vi "Phasor Compute Gated Decay (Tolerance).vi"(4 "Non Dirac IRF or non-0 lifetime":bool, 6 "tolerance":dbl, 8 "Error In":errorcluster, 9 "IRF Period":dbl, 10 "Gate & Decay Parameters Array":T1[](array[typedef]) {"A" format="%#_4g"; "s" format="%#_4g"; "sF" format="%#_4g"; "sR" format="%#_4g"; "t_i" format="%#_4g"; "t_0" format="%#_4g"; "tau" format="%#_4g"; "T" format="%#_4g"; "W" format="%#_4g"}, 11 "Time Points {t_i}":dbl[](array[numeric])) -> (0 "Error Out":errorcluster, 3 "{F(t_i)}":dbl[](array[numeric]))   [LabVIEW 2021, in "Phasor.lvlib"]
uses:
  Phasor.lvlib
  Phasor Gate & Decay Parameters.ctl
  Phasor Gate Type.ctl
  Phasor IRF Model.ctl
  Graphs/XY Graph/XY Graph Plot Data.ctl
  Phasor Abort Parallel Computation.vi
  1D Quadrature Integrand for Gated Decay.vi
  <vilib>/Utility/error.llb/Error Cluster From Error Code.vi
  <vilib>/ErrorRing/Error Ring.xnode
  Math/Math.lvlib
  Utilities/Utilities.lvlib
  Graphs/XY Graph/XY Graph Add-Ons.lvlib
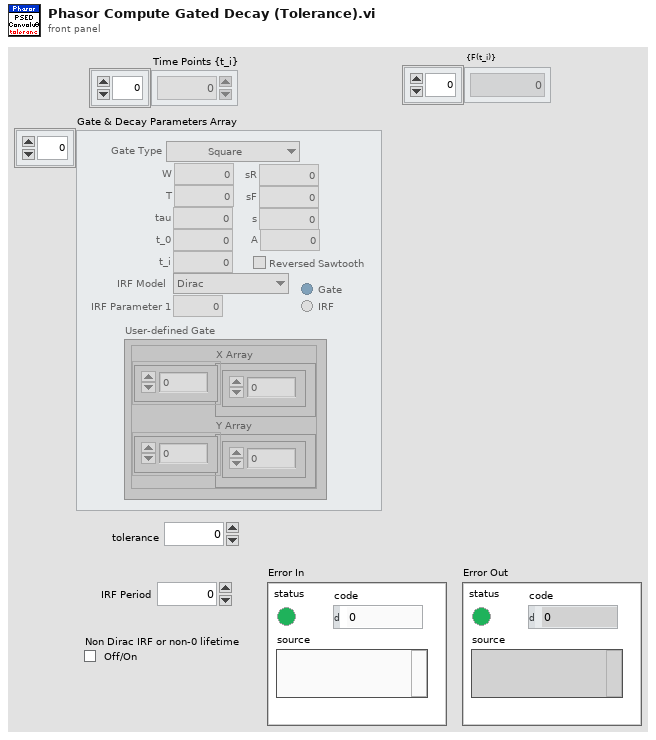
[diagram p1: front panel]
types:
  T1 = typedef "Phasor.lvlib/Phasor Gate & Decay Parameters.ctl" = cluster{"W":dbl, "T":dbl, "tau":dbl, "t_0":dbl, "Gate Type":T2, "t_i":dbl, "sR":dbl, "sF":dbl, "s":dbl, "Reversed Sawtooth":bool, "IRF Model":T3, "IRF Parameter 1":dbl, "User-defined Gate":T4, "Type of User-defined Function":enum32{"Gate", "IRF"}, "A":dbl}
  T2 = typedef "Phasor.lvlib/Phasor Gate Type.ctl" = enum16{"Square", "Finite Edge Square", "Finite Edge, Tilted Top Square", "Triangle", "Sawtooth", "User-defined"}
  T3 = typedef "Phasor.lvlib/Phasor IRF Model.ctl" = enum16{"Dirac", "Exponential"}
  T4 = typedef "XY Graph Add-Ons.lvlib/XY Graph Plot Data.ctl" = cluster{"X Array":dbl[], "Y Array":dbl[]}
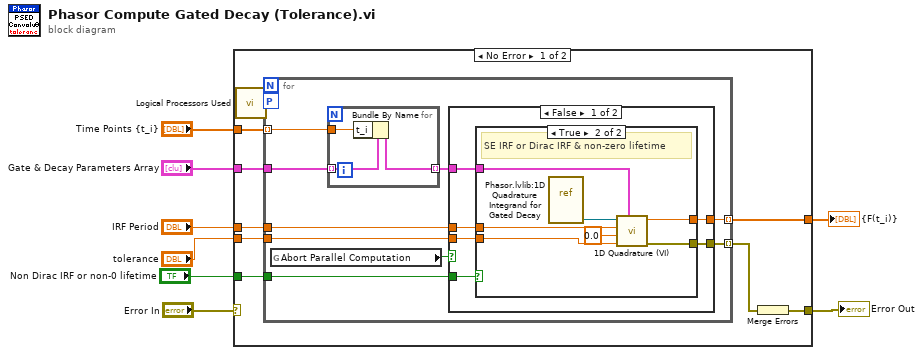
[diagram p0: block diagram]
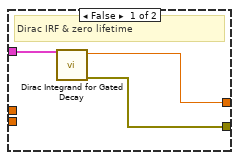
[diagram p2: hidden frame]
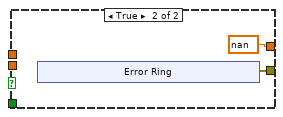
[diagram p3: hidden frame]
diagram:
  n1 = case shown="No Error" "Error In" {
    selector: "Error In" -> [_ w52]
    tunnel: "Non Dirac IRF or non-0 lifetime" -> [w17 _]
    tunnel: "IRF Period" -> [w16 _]
    tunnel: "tolerance" -> [w15 _]
    tunnel: [w14 _] -> w5
    tunnel: "Gate & Decay Parameters Array" -> [w13 _]
    tunnel: "Time Points {t_i}" -> [w12 _]
    tunnel: [w10 w52] -> w1
    frame No Error {
      n2 = call "Logical Processors Used.vi"() -> ("# Logical Processor Used"=w9:i32)  [unwired: 6 in]
      n3 = for {
        tunnel: w12 -> [w22] mode=indexing
        tunnel: w13 -> [w21]
        tunnel: [w26] -> w14 mode=indexing
        workers-P: w9 -> [_]
        tunnel: [w24] -> w11 mode=indexing
        tunnel: w15 -> [w25]
        tunnel: w16 -> [w23]
        tunnel: w17 -> [w19]
        n4 = global read "Phasor Abort Parallel Computation.vi" "Abort Parallel Computation"() -> (w18:bool)
        n5 = for {
          tunnel: w22 -> [w51]
          tunnel: w21 -> [w50] mode=indexing
          tunnel: [w49] -> w20 mode=indexing
          n6 = Bundle By Name(cluster=w50, "t_i"=w51) -> (w49:T1)
        }
        n7 = case shown="False" w18 {
          tunnel: w20 -> [w32 _]
          tunnel: [w31 nan ("result")] -> w26
          tunnel: [w30 w43] -> w24
          tunnel: w25 -> [w29 _]
          tunnel: w23 -> [w28 _]
          tunnel: w19 -> [w27 _]
          frame False {
            n8 = case shown="True" w27 {
              tunnel: [w34 w42] -> w31
              tunnel: w32 -> [w35 w41]
              tunnel: [w33 w40] -> w30
              tunnel: w29 -> [_ w39]
              tunnel: w28 -> [_ w37]
              frame False {
                # "Dirac IRF & zero lifetime"
                n9 = call "Dirac Integrand for Gated Decay.vi"("data"=w35) -> ("Error Out"=w33:errorcluster, "F(X)"=w34:dbl)  [unwired: 9 in]
              }
              frame True {
                # "SE IRF or Dirac IRF & non-zero lifetime"
                n10 = vi-ref "Phasor.lvlib:1D Quadrature Integrand for Gated Decay.vi"() -> (w36:refnum<vi>)
                n11 = call "1D Quadrature (VI).vi"("data"=w41, "tolerance"=w39, "lower limit"=0.0, "upper limit"=w37, "integrand"=w36) -> ("Error Out"=w40:errorcluster, "result"=w42:dbl)  [unwired: 5 in]
              }
            }
          }
          frame True {
            n12 = xnode "Error Ring"() -> ("error out"=w43:errorcluster)
          }
        }
      }
      n13 = Merge Errors(w11) -> (w10:errorcluster)
    }
    frame Error {
    }
  }
  "{F(t_i)}" <- w5
  "Error Out" <- w1
